vi "Computer GPS.vi"(10 "VISA resource name":refnum<visa-resource-name>) -> ()   [LabVIEW 2010]
uses:
  UDP 3.ctl
  UDP3GLOB.vi
  <instrlib>/u-blox 5 Series/u-blox 5 Series.lvlib
panel:
  out "output cluster":T1
  out "Valid Satalites":bool
  in  "Reset (False)":bool
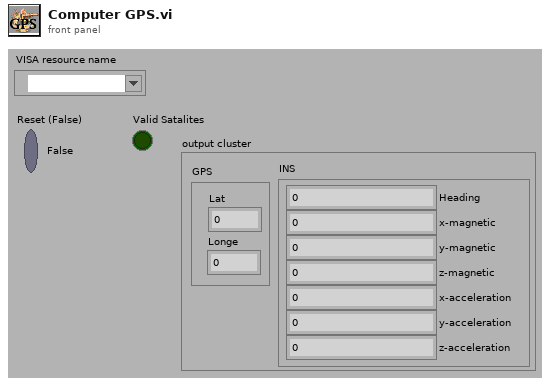
[diagram p1: front panel]
types:
  T1 = typedef "UDP 3.ctl" = cluster{"GPS":cluster{"Lat":dbl, "Longe":dbl}, "INS":cluster{"Heading":dbl, "x-magnetic":dbl, "y-magnetic":dbl, "z-magnetic":dbl, "x-acceleration":dbl, "y-acceleration":dbl, "z-acceleration":dbl}}
  T2 = cluster{"Timestamp":timestamp, "Latitude":dbl, "Longitude":dbl}[]
  T3 = cluster{"Timestamp":timestamp, "Latitude":dbl, "Longitude":dbl}
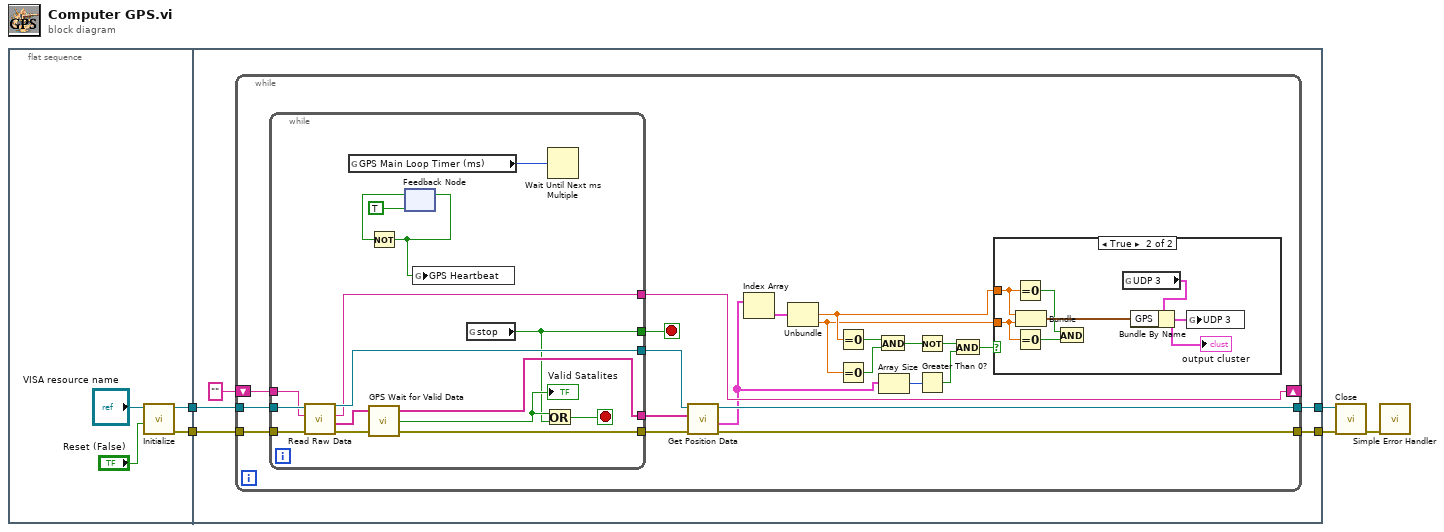
[diagram p0: block diagram]
diagram:
  n1 = flat-sequence {
    tunnel: [w7] -> w2
    tunnel: [w6] -> w1
    tunnel: [w13] -> w4
    tunnel: [w14] -> w5
    tunnel: w1 -> [w10]
    tunnel: w2 -> [w11]
    frame #0 {
      n2 = call <instrlib>:"Initialize.vi"("Reset (False)"="Reset (False)", "VISA resource name"="VISA resource name") -> ("error out"=w6:errorcluster, "VISA resource name out"=w7:refnum<visa-resource-name>)  [unwired: 8 in]
    }
    frame #1 {
      n3 = while {
        shift-right: [w32] -> _
        shift-left: "" ("Remaining Partial Sentence") -> [w35]
        tunnel: w11 -> [w34]
        tunnel: w10 -> [w33]
        tunnel: [w26] -> w13
        tunnel: [w25] -> w14
        stop <- w23 stop-if-true
        n4 = while {
          tunnel: [w58] -> w31
          tunnel: w34 -> [w57]
          tunnel: w33 -> [w56]
          tunnel: w35 -> [w54]
          tunnel: [w51] -> w30
          tunnel: [w47] -> w23
          tunnel: [w50] -> w29
          tunnel: [w49] -> w32
          stop <- w55 stop-if-true
          n5 = call <instrlib>:"Read Raw Data.vi"("error in (no error)"=w56, "Previous Partial Sentence"=w54, "VISA resource name"=w57) -> ("error out"=w53:errorcluster, "Complete NMEA Sentences"=w52:string[], "Remaining Partial Sentence"=w49:string, "VISA resource name out"=w58:refnum<visa-resource-name>)  [unwired: 5 in]
          n6 = global read "UDP3GLOB.vi" "GPS Main Loop Timer (ms)"() -> (w43:u32)
          n7 = call "GPS Wait for Valid Data.vi"("error in (no error)"=w53, "Completed NMEA Sentences"=w52) -> ("error out"=w50:errorcluster, "Valid Data"=w48:bool, "Complete NMEA Sentences (Copy)"=w51:string[])  [unwired: 1 in]
          "Valid Satalites" <- w48
          n8 = feedback #1(TRUE) -> (w45:bool)
          n9 = Not(x=w45) -> (.not. x?=w44:bool)
          n10 = feedback-in #1(w44) -> ()
          n11 = global write "UDP3GLOB.vi" "GPS Heartbeat"(w44) -> ()
          n12 = global read "UDP3GLOB.vi" "stop"() -> (w47:bool)
          n13 = Or(x=w48, y=w47) -> (x .or. y?=w55:bool)
          n14 = Wait Until Next ms Multiple(millisecond multiple=w43) -> ()  [unwired: 1 out]
        }
        n15 = call <instrlib>:"Get Position Data.vi"("error in (no error)"=w29, "Complete NMEA Sentences"=w30, "VISA resource name"=w31) -> ("error out"=w25:errorcluster, "Position Data"=w24:T2, "VISA resource name out"=w26:refnum<visa-resource-name>)  [unwired: 5 in, 1 out]
        n16 = Index Array(array=w24) -> (element=w27:T3)  [unwired: 1 in]
        n17 = Unbundle(w27) -> ("Latitude"=w19:dbl, "Longitude"=w18:dbl)  [unwired: 1 out]
        n18 = Equal To 0?(x=w19) -> (x = 0?=w21:bool)
        n19 = Equal To 0?(x=w18) -> (x = 0?=w20:bool)
        n20 = And(x=w21, y=w20) -> (x .and. y?=w16:bool)
        n21 = Array Size(array=w24) -> (size(s)=w28:i32)
        n22 = Not(x=w16) -> (.not. x?=w15:bool)
        n23 = Greater Than 0?(x=w28) -> (x > 0?=w22:bool)
        n24 = And(x=w15, y=w22) -> (x .and. y?=w17:bool)
        n25 = case shown="True" w17 {
          tunnel: w18 -> [_ w40]
          tunnel: w19 -> [_ w39]
          frame False {
          }
          frame True {
            n26 = Equal To 0?(x=w39) -> (x = 0?=w37:bool)
            n27 = Equal To 0?(x=w40) -> (x = 0?=w38:bool)
            n28 = Bundle("Latitude"=w39, "Longitude"=w40) -> (w42:cluster{"Latitude":dbl, "Longitude":dbl})  [unwired: 1 in]
            n29 = And(x=w37, y=w38) -> ()  [unwired: 1 out]
            n30 = global read "UDP3GLOB.vi" "UDP 3"() -> (w36:T1)
            n31 = Bundle By Name(cluster=w36, "GPS"=w42) -> (w41:T1)
            "output cluster" <- w41
            n32 = global write "UDP3GLOB.vi" "UDP 3"(w41) -> ()
          }
        }
      }
    }
  }
  n33 = call <instrlib>:"Close.vi"("error in (no error)"=w5, "VISA resource name"=w4) -> ("error out"=w3:errorcluster)  [unwired: 9 in]
  n34 = call <vilib>:"Simple Error Handler.vi"("error in (no error)"=w3) -> ()  [unwired: 4 in, 5 out]
